vi "Read Operator Joystick.vi"   [LabVIEW 2020]
uses:
  <vilib>/Rock Robotics/Network Tables/NT Write Boolean Array.vi
  <vilib>/Rock Robotics/Network Tables/NT Write Numeric Array.vi
  Framework/Robot Global Data.vi
panel:
  # "READ OPERATOR JOYSTICK"
types:
  T1 = enum16{"0", "1", "2", "3", "4", "5", "6", "7", "8", "9", "10", "11"}
  T2 = typedef "WPI_JoystickDevRef.ctl" = cluster{"Device":T3}
  T3 = typedef "WPI_JoystickDeviceEnum.ctl" = enum16{"USB 0", "USB 1", "USB 2", "USB 3", "USB 4", "USB 5"}
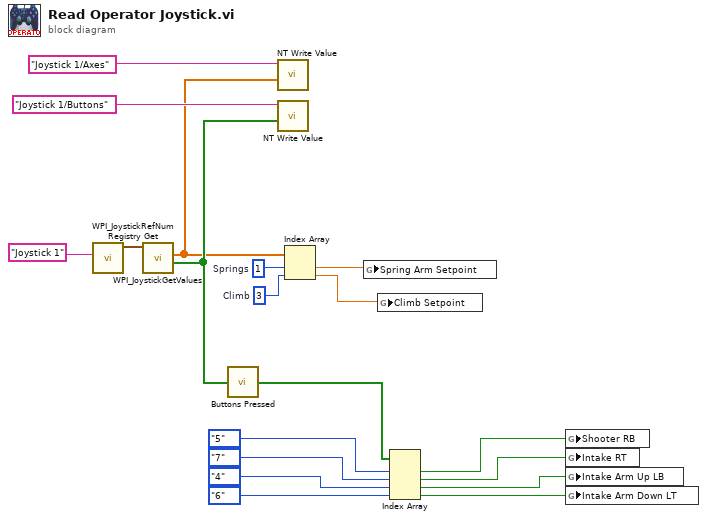
[diagram p0: block diagram]
diagram:
  w12 = 1  # Springs
  w11 = 3  # Climb
  n1 = call <vilib>:"WPI_JoystickRefNum Registry Get.vi"("refnum name"="Joystick 1") -> ("JoystickDevRef"=w18:T2)  [unwired: 1 in, 9 out]
  n2 = call <vilib>:"WPI_JoystickGetValues.vi"("JoystickDevRef"=w18) -> ("Buttons"=w15:bool[], "Axes"=w14:dbl[])  [unwired: 6 in, 3 out]
  n3 = call "Buttons Pressed.vi"("Button Values"=w15) -> ("Button Presses"=w17:bool[])
  n4 = call-poly <vilib>:"NT Write Value.vi"("Numeric Array"=w14, "Name"="Joystick 1/Axes") -> ()  [unwired: 9 in, 1 out]
  n5 = call-poly <vilib>:"NT Write Value.vi"("Boolean Array"=w15, "Name"="Joystick 1/Buttons") -> ()  [unwired: 9 in, 1 out]
  n6 = Index Array(array=w14, index #1=w12, index #2=w11) -> (element #1=w3:dbl, element #2=w2:dbl)
  n7 = global write "Robot Global Data.vi" "Spring Arm Setpoint"(w3) -> ()
  n8 = global write "Robot Global Data.vi" "Climb Setpoint"(w2) -> ()
  n9 = Index Array(array=w17, index #1=T1."5", index #2=T1."7", index #3=T1."4", index #4=T1."6") -> (element #1=w6:bool, element #2=w5:bool, element #3=w4:bool, element #4=w1:bool)
  n10 = global write "Robot Global Data.vi" "Shooter RB"(w6) -> ()
  n11 = global write "Robot Global Data.vi" "Intake RT"(w5) -> ()
  n12 = global write "Robot Global Data.vi" "Intake Arm Up LB"(w4) -> ()
  n13 = global write "Robot Global Data.vi" "Intake Arm Down LT"(w1) -> ()
